vi "Player Info.vi"(8 "Victory Speech":string, 9 "Name":string, 11 "Square in":refnum<class "Square.lvclass">) -> (3 "Square out":refnum<class "Square.lvclass">)   [LabVIEW 2015, in "Square.lvclass"]
uses:
  Square.lvclass
panel:
  # "Set default values for these two string controls"
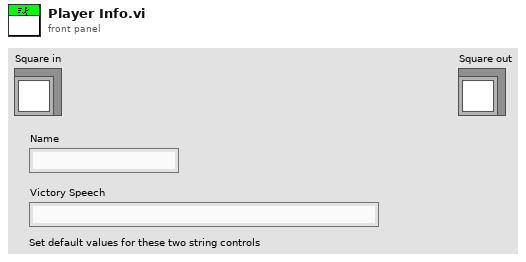
[diagram p1: front panel]
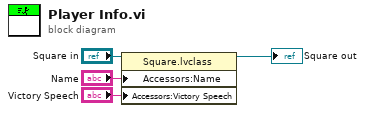
[diagram p0: block diagram]
diagram:
  n1 = property class="Square.lvclass"(reference="Square in", "Accessors:Name"="Name", "Accessors:Victory Speech"="Victory Speech") -> (reference out=→"Square out":refnum<class "Square.lvclass">)  [unwired: 1 in, 1 out]
